vi "Write.vi"(8 "error in (no error)":errorcluster, 10 "write data":T1, 11 "ModbusSp in":refnum<class "ModbusSp.lvclass">) -> (0 "error out":errorcluster, 3 "ModbusSp out":refnum<class "ModbusSp.lvclass">)   [LabVIEW 2019, in "ModbusSp.lvclass"]
uses:
  ModbusSp.lvclass
  WriteData.ctl
  ModbusSp.lvclass/ModbusSp.ctl
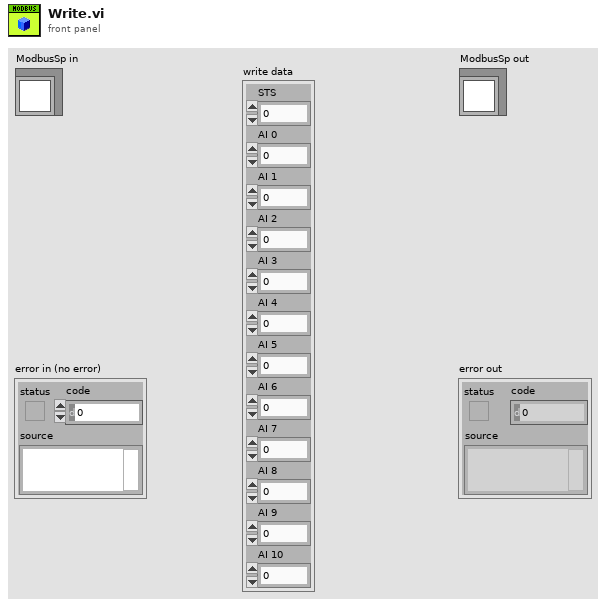
[diagram p1: front panel]
types:
  T1 = typedef "ModbusSp.lvclass/WriteData.ctl" = cluster{"STS":u16, "AI 0":sgl, "AI 1":sgl, "AI 2":sgl, "AI 3":sgl, "AI 4":sgl, "AI 5":sgl, "AI 6":sgl, "AI 7":sgl, "AI 8":sgl, "AI 9":sgl, "AI 10":sgl}
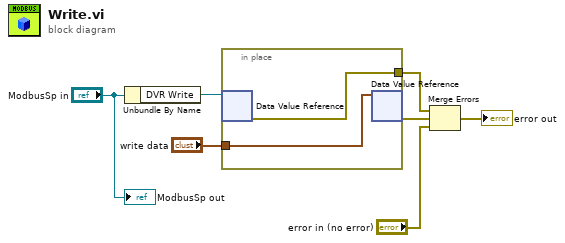
[diagram p0: block diagram]
diagram:
  n1 = Unbundle By Name("ModbusSp in") -> ("DVR Write"=w5:refnum<data-value>)
  n2 = in-place {
    in-place-border: [w9] -> w2
    in-place-border: "write data" -> [w8]
    n3 = in-place-dvr #1(w5) -> (w9:errorcluster)  [unwired: 1 out]
    n4 = in-place-dvr #1(w8) -> (w3:errorcluster)  [unwired: 1 out]
  }
  n5 = Merge Errors(w2, w3, "error in (no error)") -> (→"error out":errorcluster)
  "ModbusSp out" <- "ModbusSp in"
